vi "DisabelConnectButton.vi"(8 "error in (no error)":errorcluster, 10 "Connect button Disabled":T1(ring), 11 "TCP_Client in":refnum<class "TCP_Client.lvclass">) -> (0 "error out":errorcluster, 3 "TCP_Client out":refnum<class "TCP_Client.lvclass">)   [LabVIEW 2023, in "TCP_Client.lvlib" / "TCP_Client.lvclass"]
uses:
  TCP_Client.lvclass
  TCP_Client.lvclass/TCP_Client.ctl
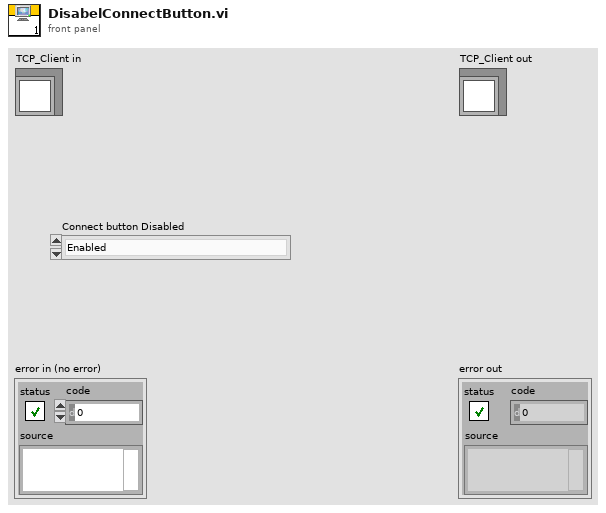
[diagram p1: front panel]
types:
  T1 = enum8{"Enabled", "Disabled", "Disabled and Grayed Out"}
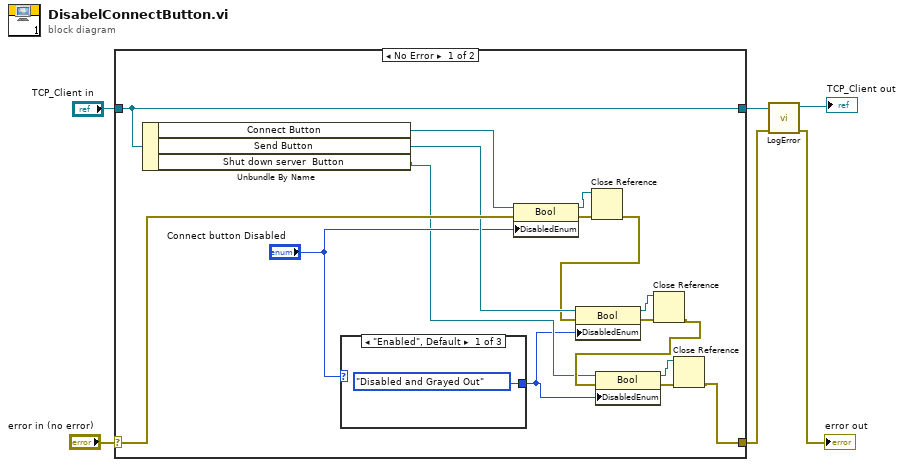
[diagram p0: block diagram]
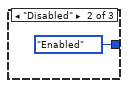
[diagram p2: hidden frame]
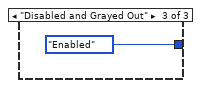
[diagram p3: hidden frame]
diagram:
  n1 = case shown="No Error" "error in (no error)" {
    selector: "error in (no error)" -> [w21 w27]
    tunnel: [w7 w27] -> w2
    tunnel: [w18 w26] -> w4
    tunnel: "TCP_Client in" -> [w18 w26]
    frame No Error {
      n2 = Unbundle By Name(w18) -> ("Connect Button"=w22:refnum<vi>, "Send Button"=w15:refnum<vi>, "Shut down server  Button"=w9:refnum<vi>)
      n3 = case shown="\"Enabled\", Default" "Connect button Disabled" {
        tunnel: [T1."Disabled and Grayed Out" ("Disabled") T1."Enabled" ("Disabled") T1."Enabled" ("Disabled")] -> w8
        frame "Enabled", Default {
        }
        frame "Disabled" {
        }
        frame "Disabled and Grayed Out" {
        }
      }
      n4 = property class="Bool"(reference=w22, error in=w21, "DisabledEnum"="Connect button Disabled") -> (reference out=w19:refnum<vi>, error out=w20:errorcluster)
      n5 = Close Reference(reference=w19, error in (no error)=w20) -> (error out=w14:errorcluster)
      n6 = property class="Bool"(reference=w15, error in=w14, "DisabledEnum"=w8) -> (reference out=w17:refnum<vi>, error out=w16:errorcluster)
      n7 = Close Reference(reference=w17, error in (no error)=w16) -> (error out=w10:errorcluster)
      n8 = property class="Bool"(reference=w9, error in=w10, "DisabledEnum"=w8) -> (reference out=w11:refnum<vi>, error out=w12:errorcluster)
      n9 = Close Reference(reference=w11, error in (no error)=w12) -> (error out=w7:errorcluster)
    }
    frame Error {
    }
  }
  n10 = call "LogError.vi"("error in (no error)"=w2, "TCP_Client in"=w4) -> ("error out"=→"error out":errorcluster, "TCP_Client out"=→"TCP_Client out":refnum<class "TCP_Client.lvclass">)  [unwired: 8 in]
